vi "Option Selection.vi"(0 "GEA2 Reference In":refnum<k24>, 5 "Options":T2, 7 "Change":T1, 9 "Change All?":bool, 11 "Error In":errorcluster) -> (4 "GEA2 Reference Out":refnum<k24>, 15 "Error Out":errorcluster)   [LabVIEW 2016, in "2015 VA Washer.lvlib"]
doc: "Use this VI to select options on the HEUI or LEUI. These options are selected through their respective ERDs, not by a button press or knob turn."
uses:
  Projects/2015 VA Washer.lvlib
  C:/Automation/DLLs/PC Dot Net/GeaCommunication.dll
  Common/LabVIEW GEA2 Toolkit/LabVIEW_GEA2_Toolkit.lvlibp/type defs/Source_Destination.ctl
  Common/LabVIEW GEA2 Toolkit/LabVIEW_GEA2_Toolkit.lvlibp/type defs/ERD Write Data In.ctl
  Common/LabVIEW GEA2 Toolkit/LabVIEW_GEA2_Toolkit.lvlibp/type defs/Data Type.ctl
  Common/LabVIEW GEA2 Toolkit/LabVIEW_GEA2_Toolkit.lvlibp
panel:
  in  "Standalone?":bool
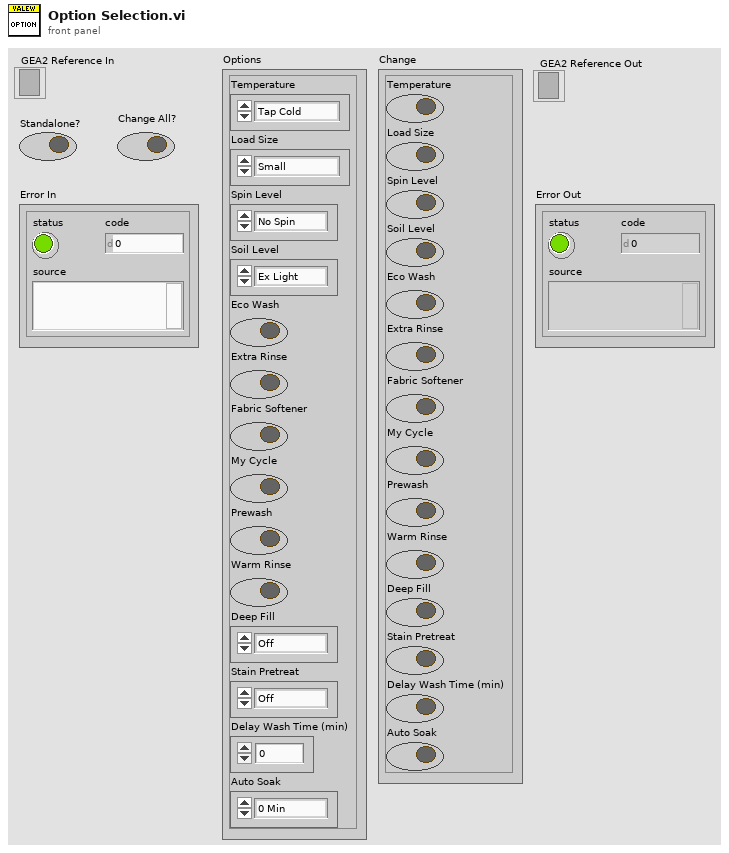
[diagram p1: front panel]
types:
  T1 = cluster{"Temperature":bool, "Load Size":bool, "Spin Level":bool, "Soil Level":bool, "Eco Wash":bool, "Extra Rinse":bool, "Fabric Softener":bool, "My Cycle":bool, "Prewash":bool, "Warm Rinse":bool, "Deep Fill":bool, "Stain Pretreat":bool, "Delay Wash Time (min)":bool, "Auto Soak":bool}
  T2 = cluster{"Temperature":enum16{"Tap Cold", "Cold", "Cool", "Colors", "Warm", "Hot"}, "Load Size":enum16{"Small", "Medium", "Large", "Super", "Precise Fill (Super Plus)"}, "Spin Level":enum16{"No Spin", "Normal", "More", "Max"}, "Soil Level":enum16{"Ex Light", "Light", "Normal", "Heavy", "Ex Heavy"}, "Eco Wash":bool, "Extra Rinse":bool, "Fabric Softener":bool, "My Cycle":bool, "Prewash":bool, "Warm Rinse":bool, "Deep Fill":enum16{"Off", "Incremental", "Max"}, "Stain Pretreat":enum16{"Off", "Tomato", "Wine", "Blood", "Grass", "Dirt"}, "Delay Wash Time (min)":u16, "Auto Soak":enum16{"0 Min", "15 Min", "30 Min", "60 Min", "2 Hr"}}
  T3 = typedef "LabVIEW_GEA2_Toolkit.lvlibp/Source_Destination.ctl" = cluster{"Source":u8, "Destination":u8}
  T4 = enum16{"Tap Cold", "Cold", "Cool", "Colors", "Warm", "Hot"}
  T5 = typedef "LabVIEW_GEA2_Toolkit.lvlibp/ERD Write Data In.ctl" = cluster{"ERD Number":u16, "Data Type":T6, "Data":string}
  T6 = typedef "LabVIEW_GEA2_Toolkit.lvlibp/Data Type.ctl" = enum16{"string", "boolean", "uint8_t", "uint16_t", "uint32_t", "uint64_t", "int8_t", "int16_t", "int32_t", "int64_t"}
  T7 = enum16{"Small", "Medium", "Large", "Super", "Precise Fill (Super Plus)"}
  T8 = enum16{"Ex Light", "Light", "Normal", "Heavy", "Ex Heavy"}
  T9 = enum16{"Off", "Tomato", "Wine", "Blood", "Grass", "Dirt"}
  T10 = enum16{"0 Min", "15 Min", "30 Min", "60 Min", "2 Hr"}
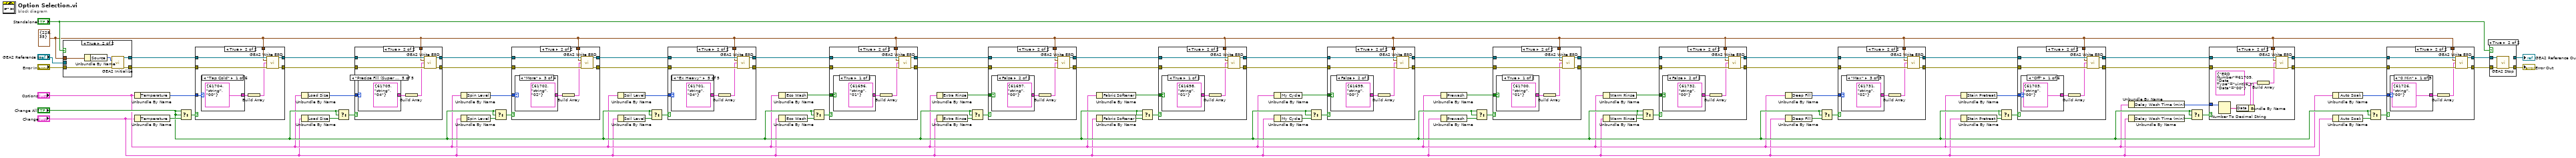
[diagram p0: block diagram]
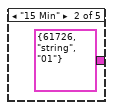
[diagram p4: hidden frame]
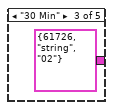
[diagram p5: hidden frame]
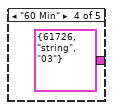
[diagram p6: hidden frame]
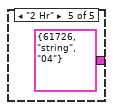
[diagram p7: hidden frame]
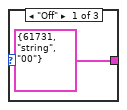
[diagram p9: hidden frame]
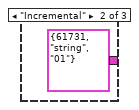
[diagram p10: hidden frame]
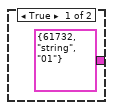
[diagram p12: hidden frame]
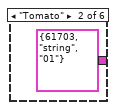
[diagram p14: hidden frame]
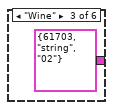
[diagram p15: hidden frame]
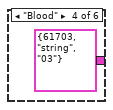
[diagram p16: hidden frame]
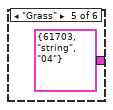
[diagram p17: hidden frame]
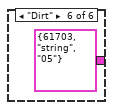
[diagram p18: hidden frame]
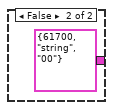
[diagram p20: hidden frame]
diagram:
  w8 = T3 {"Source"=228, "Destination"=35} ("GEA Inputs")
  n1 = case shown="True" "Standalone?" {
    tunnel: "Error In" -> [w82 w88]
    tunnel: [w82 w87] -> w76
    tunnel: "GEA2 Reference In" -> [w83 _]
    tunnel: [w83 w86] -> w81
    tunnel: w8 -> [_ w84]
    frame False {
    }
    frame True {
      n2 = Unbundle By Name(w84) -> ("Source"=w85:u8)
      n3 = call "GEA2 Initialize.vi"("Source Address"=w85, "error in"=w88) -> ("GEA2 Reference Out"=w86:refnum<k24>, "error out"=w87:errorcluster)  [unwired: 11 in, 1 out]
    }
  }
  n4 = Unbundle By Name("Options") -> ("Temperature"=w73:T4)
  n5 = Unbundle By Name("Change") -> ("Temperature"=w74:bool)
  n6 = Select(t="Change All?", s="Change All?", f=w74) -> (s? t:f=w72:bool)
  n7 = case shown="True" w72 {
    tunnel: w81 -> [w90 w98]
    tunnel: w76 -> [w89 w97]
    tunnel: w8 -> [_ w96]
    tunnel: [w90 w94] -> w68
    tunnel: [w89 w93] -> w67
    tunnel: w73 -> [_ w91]
    frame False {
    }
    frame True {
      n8 = case shown="\"Tap Cold\"" w91 {
        tunnel: [T5 {"ERD Number"=61704, "Data Type"=enum."string", "Data"="00"} ("ERD Write Data In") T5 {"ERD Number"=61704, "Data Type"=enum."string", "Data"="01"} ("ERD Write Data In") T5 {"ERD Number"=61704, "Data Type"=enum."string", "Data"="02"} ("ERD Write Data In") T5 {"ERD Number"=61704, "Data Type"=enum."string", "Data"="03"} ("ERD Write Data In") T5 {"ERD Number"=61704, "Data Type"=enum."string", "Data"="04"} ("ERD Write Data In") T5 {"ERD Number"=61704, "Data Type"=enum."string", "Data"="05"} ("ERD Write Data In")] -> w92
        frame "Tap Cold" {
        }
        frame "Cold" {
        }
        frame "Cool" {
        }
        frame "Colors" {
        }
        frame "Warm" {
        }
        frame "Hot" {
        }
      }
      n9 = Build Array(w92) -> (w95:T5[])
      n10 = call "GEA2 Write ERD.vi"("GEA2 Reference In"=w98, "GEA Inputs"=w96, "Write ERD List"=w95, "Error In"=w97) -> ("GEA2 Reference Out"=w94:refnum<k24>, "Error Out"=w93:errorcluster)  [unwired: 9 in, 1 out]
    }
  }
  n11 = Unbundle By Name("Options") -> ("Load Size"=w70:T7)
  n12 = Unbundle By Name("Change") -> ("Load Size"=w69:bool)
  n13 = Select(t="Change All?", s="Change All?", f=w69) -> (s? t:f=w71:bool)
  n14 = case shown="True" w71 {
    tunnel: w68 -> [w106 w114]
    tunnel: w67 -> [w105 w113]
    tunnel: w8 -> [_ w112]
    tunnel: [w106 w109] -> w63
    tunnel: [w105 w108] -> w62
    tunnel: w70 -> [_ w107]
    frame False {
    }
    frame True {
      n15 = case shown="\"Precise Fill (Super Plus)\"" w107 {
        tunnel: [T5 {"ERD Number"=61705, "Data Type"=enum."string", "Data"="00"} ("ERD Write Data In") T5 {"ERD Number"=61705, "Data Type"=enum."string", "Data"="01"} ("ERD Write Data In") T5 {"ERD Number"=61705, "Data Type"=enum."string", "Data"="02"} ("ERD Write Data In") T5 {"ERD Number"=61705, "Data Type"=enum."string", "Data"="03"} ("ERD Write Data In") T5 {"ERD Number"=61705, "Data Type"=enum."string", "Data"="04"} ("ERD Write Data In")] -> w111
        frame "Small" {
        }
        frame "Medium" {
        }
        frame "Large" {
        }
        frame "Super" {
        }
        frame "Precise Fill (Super Plus)" {
        }
      }
      n16 = Build Array(w111) -> (w110:T5[])
      n17 = call "GEA2 Write ERD.vi"("GEA2 Reference In"=w114, "GEA Inputs"=w112, "Write ERD List"=w110, "Error In"=w113) -> ("GEA2 Reference Out"=w109:refnum<k24>, "Error Out"=w108:errorcluster)  [unwired: 9 in, 1 out]
    }
  }
  n18 = Unbundle By Name("Options") -> ("Spin Level"=w65:enum16{"No Spin", "Normal", "More", "Max"})
  n19 = Unbundle By Name("Change") -> ("Spin Level"=w66:bool)
  n20 = Select(t="Change All?", s="Change All?", f=w66) -> (s? t:f=w64:bool)
  n21 = case shown="True" w64 {
    tunnel: w63 -> [w121 w129]
    tunnel: w62 -> [w120 w128]
    tunnel: w8 -> [_ w127]
    tunnel: [w121 w124] -> w58
    tunnel: [w120 w123] -> w57
    tunnel: w65 -> [_ w122]
    frame False {
    }
    frame True {
      n22 = case shown="\"More\"" w122 {
        tunnel: [T5 {"ERD Number"=61702, "Data Type"=enum."string", "Data"="00"} ("ERD Write Data In") T5 {"ERD Number"=61702, "Data Type"=enum."string", "Data"="01"} ("ERD Write Data In") T5 {"ERD Number"=61702, "Data Type"=enum."string", "Data"="02"} ("ERD Write Data In") T5 {"ERD Number"=61702, "Data Type"=enum."string", "Data"="03"} ("ERD Write Data In")] -> w126
        frame "No Spin" {
        }
        frame "Normal" {
        }
        frame "More" {
        }
        frame "Max" {
        }
      }
      n23 = Build Array(w126) -> (w125:T5[])
      n24 = call "GEA2 Write ERD.vi"("GEA2 Reference In"=w129, "GEA Inputs"=w127, "Write ERD List"=w125, "Error In"=w128) -> ("GEA2 Reference Out"=w124:refnum<k24>, "Error Out"=w123:errorcluster)  [unwired: 9 in, 1 out]
    }
  }
  n25 = Unbundle By Name("Options") -> ("Soil Level"=w60:T8)
  n26 = Unbundle By Name("Change") -> ("Soil Level"=w59:bool)
  n27 = Select(t="Change All?", s="Change All?", f=w59) -> (s? t:f=w61:bool)
  n28 = case shown="True" w61 {
    tunnel: w58 -> [w135 w143]
    tunnel: w57 -> [w134 w142]
    tunnel: w8 -> [_ w141]
    tunnel: [w135 w138] -> w53
    tunnel: [w134 w137] -> w52
    tunnel: w60 -> [_ w136]
    frame False {
    }
    frame True {
      n29 = case shown="\"Ex Heavy\"" w136 {
        tunnel: [T5 {"ERD Number"=61701, "Data Type"=enum."string", "Data"="00"} ("ERD Write Data In") T5 {"ERD Number"=61701, "Data Type"=enum."string", "Data"="01"} ("ERD Write Data In") T5 {"ERD Number"=61701, "Data Type"=enum."string", "Data"="02"} ("ERD Write Data In") T5 {"ERD Number"=61701, "Data Type"=enum."string", "Data"="03"} ("ERD Write Data In") T5 {"ERD Number"=61701, "Data Type"=enum."string", "Data"="04"} ("ERD Write Data In")] -> w140
        frame "Ex Light" {
        }
        frame "Light" {
        }
        frame "Normal" {
        }
        frame "Heavy" {
        }
        frame "Ex Heavy" {
        }
      }
      n30 = Build Array(w140) -> (w139:T5[])
      n31 = call "GEA2 Write ERD.vi"("GEA2 Reference In"=w143, "GEA Inputs"=w141, "Write ERD List"=w139, "Error In"=w142) -> ("GEA2 Reference Out"=w138:refnum<k24>, "Error Out"=w137:errorcluster)  [unwired: 9 in, 1 out]
    }
  }
  n32 = Unbundle By Name("Options") -> ("Eco Wash"=w55:bool)
  n33 = Unbundle By Name("Change") -> ("Eco Wash"=w56:bool)
  n34 = Select(t="Change All?", s="Change All?", f=w56) -> (s? t:f=w54:bool)
  n35 = case shown="True" w54 {
    tunnel: w53 -> [w150 w158]
    tunnel: w52 -> [w149 w157]
    tunnel: w8 -> [_ w156]
    tunnel: [w150 w153] -> w47
    tunnel: [w149 w152] -> w48
    tunnel: w55 -> [_ w151]
    frame False {
    }
    frame True {
      n36 = case shown="True" w151 {
        tunnel: [T5 {"ERD Number"=61696, "Data Type"=enum."string", "Data"="01"} ("ERD Write Data In") T5 {"ERD Number"=61696, "Data Type"=enum."string", "Data"="00"} ("ERD Write Data In")] -> w155
        frame True {
        }
        frame False {
        }
      }
      n37 = Build Array(w155) -> (w154:T5[])
      n38 = call "GEA2 Write ERD.vi"("GEA2 Reference In"=w158, "GEA Inputs"=w156, "Write ERD List"=w154, "Error In"=w157) -> ("GEA2 Reference Out"=w153:refnum<k24>, "Error Out"=w152:errorcluster)  [unwired: 9 in, 1 out]
    }
  }
  n39 = Unbundle By Name("Options") -> ("Extra Rinse"=w50:bool)
  n40 = Unbundle By Name("Change") -> ("Extra Rinse"=w49:bool)
  n41 = Select(t="Change All?", s="Change All?", f=w49) -> (s? t:f=w51:bool)
  n42 = case shown="True" w51 {
    tunnel: w47 -> [w162 w170]
    tunnel: w48 -> [w161 w169]
    tunnel: w8 -> [_ w168]
    tunnel: [w162 w165] -> w43
    tunnel: [w161 w164] -> w42
    tunnel: w50 -> [_ w163]
    frame False {
    }
    frame True {
      n43 = case shown="False" w163 {
        tunnel: [T5 {"ERD Number"=61697, "Data Type"=enum."string", "Data"="01"} ("ERD Write Data In") T5 {"ERD Number"=61697, "Data Type"=enum."string", "Data"="00"} ("ERD Write Data In")] -> w167
        frame True {
        }
        frame False {
        }
      }
      n44 = Build Array(w167) -> (w166:T5[])
      n45 = call "GEA2 Write ERD.vi"("GEA2 Reference In"=w170, "GEA Inputs"=w168, "Write ERD List"=w166, "Error In"=w169) -> ("GEA2 Reference Out"=w165:refnum<k24>, "Error Out"=w164:errorcluster)  [unwired: 9 in, 1 out]
    }
  }
  n46 = Unbundle By Name("Options") -> ("Fabric Softener"=w45:bool)
  n47 = Unbundle By Name("Change") -> ("Fabric Softener"=w46:bool)
  n48 = Select(t="Change All?", s="Change All?", f=w46) -> (s? t:f=w44:bool)
  n49 = case shown="True" w44 {
    tunnel: w43 -> [w174 w182]
    tunnel: w42 -> [w173 w181]
    tunnel: w8 -> [_ w180]
    tunnel: [w174 w177] -> w38
    tunnel: [w173 w176] -> w37
    tunnel: w45 -> [_ w175]
    frame False {
    }
    frame True {
      n50 = case shown="True" w175 {
        tunnel: [T5 {"ERD Number"=61698, "Data Type"=enum."string", "Data"="01"} ("ERD Write Data In") T5 {"ERD Number"=61698, "Data Type"=enum."string", "Data"="00"} ("ERD Write Data In")] -> w179
        frame True {
        }
        frame False {
        }
      }
      n51 = Build Array(w179) -> (w178:T5[])
      n52 = call "GEA2 Write ERD.vi"("GEA2 Reference In"=w182, "GEA Inputs"=w180, "Write ERD List"=w178, "Error In"=w181) -> ("GEA2 Reference Out"=w177:refnum<k24>, "Error Out"=w176:errorcluster)  [unwired: 9 in, 1 out]
    }
  }
  n53 = Unbundle By Name("Options") -> ("My Cycle"=w40:bool)
  n54 = Unbundle By Name("Change") -> ("My Cycle"=w39:bool)
  n55 = Select(t="Change All?", s="Change All?", f=w39) -> (s? t:f=w41:bool)
  n56 = case shown="True" w41 {
    tunnel: w38 -> [w186 w194]
    tunnel: w37 -> [w185 w193]
    tunnel: w8 -> [_ w192]
    tunnel: [w186 w189] -> w33
    tunnel: [w185 w188] -> w32
    tunnel: w40 -> [_ w187]
    frame False {
    }
    frame True {
      n57 = case shown="False" w187 {
        tunnel: [T5 {"ERD Number"=61699, "Data Type"=enum."string", "Data"="01"} ("ERD Write Data In") T5 {"ERD Number"=61699, "Data Type"=enum."string", "Data"="00"} ("ERD Write Data In")] -> w191
        frame True {
        }
        frame False {
        }
      }
      n58 = Build Array(w191) -> (w190:T5[])
      n59 = call "GEA2 Write ERD.vi"("GEA2 Reference In"=w194, "GEA Inputs"=w192, "Write ERD List"=w190, "Error In"=w193) -> ("GEA2 Reference Out"=w189:refnum<k24>, "Error Out"=w188:errorcluster)  [unwired: 9 in, 1 out]
    }
  }
  n60 = Unbundle By Name("Options") -> ("Prewash"=w35:bool)
  n61 = Unbundle By Name("Change") -> ("Prewash"=w36:bool)
  n62 = Select(t="Change All?", s="Change All?", f=w36) -> (s? t:f=w34:bool)
  n63 = case shown="True" w34 {
    tunnel: w33 -> [w198 w206]
    tunnel: w32 -> [w197 w205]
    tunnel: w8 -> [_ w204]
    tunnel: [w198 w201] -> w25
    tunnel: [w197 w200] -> w24
    tunnel: w35 -> [_ w199]
    frame False {
    }
    frame True {
      n64 = case shown="True" w199 {
        tunnel: [T5 {"ERD Number"=61700, "Data Type"=enum."string", "Data"="01"} ("ERD Write Data In") T5 {"ERD Number"=61700, "Data Type"=enum."string", "Data"="00"} ("ERD Write Data In")] -> w203
        frame True {
        }
        frame False {
        }
      }
      n65 = Build Array(w203) -> (w202:T5[])
      n66 = call "GEA2 Write ERD.vi"("GEA2 Reference In"=w206, "GEA Inputs"=w204, "Write ERD List"=w202, "Error In"=w205) -> ("GEA2 Reference Out"=w201:refnum<k24>, "Error Out"=w200:errorcluster)  [unwired: 9 in, 1 out]
    }
  }
  n67 = Unbundle By Name("Options") -> ("Warm Rinse"=w27:bool)
  n68 = Unbundle By Name("Change") -> ("Warm Rinse"=w26:bool)
  n69 = Select(t="Change All?", s="Change All?", f=w26) -> (s? t:f=w28:bool)
  n70 = case shown="True" w28 {
    tunnel: w25 -> [w210 w218]
    tunnel: w24 -> [w209 w217]
    tunnel: w8 -> [_ w216]
    tunnel: [w210 w213] -> w20
    tunnel: [w209 w212] -> w19
    tunnel: w27 -> [_ w211]
    frame False {
    }
    frame True {
      n71 = case shown="False" w211 {
        tunnel: [T5 {"ERD Number"=61732, "Data Type"=enum."string", "Data"="01"} ("ERD Write Data In") T5 {"ERD Number"=61732, "Data Type"=enum."string", "Data"="00"} ("ERD Write Data In")] -> w215
        frame True {
        }
        frame False {
        }
      }
      n72 = Build Array(w215) -> (w214:T5[])
      n73 = call "GEA2 Write ERD.vi"("GEA2 Reference In"=w218, "GEA Inputs"=w216, "Write ERD List"=w214, "Error In"=w217) -> ("GEA2 Reference Out"=w213:refnum<k24>, "Error Out"=w212:errorcluster)  [unwired: 9 in, 1 out]
    }
  }
  n74 = Unbundle By Name("Options") -> ("Deep Fill"=w22:enum16{"Off", "Incremental", "Max"})
  n75 = Unbundle By Name("Change") -> ("Deep Fill"=w23:bool)
  n76 = Select(t="Change All?", s="Change All?", f=w23) -> (s? t:f=w21:bool)
  n77 = case shown="True" w21 {
    tunnel: w20 -> [w222 w230]
    tunnel: w19 -> [w221 w229]
    tunnel: w8 -> [_ w228]
    tunnel: [w222 w225] -> w18
    tunnel: [w221 w224] -> w17
    tunnel: w22 -> [_ w223]
    frame False {
    }
    frame True {
      n78 = case shown="\"Max\"" w223 {
        tunnel: [T5 {"ERD Number"=61731, "Data Type"=enum."string", "Data"="00"} ("ERD Write Data In") T5 {"ERD Number"=61731, "Data Type"=enum."string", "Data"="01"} ("ERD Write Data In") T5 {"ERD Number"=61731, "Data Type"=enum."string", "Data"="02"} ("ERD Write Data In")] -> w227
        frame "Off" {
        }
        frame "Incremental" {
        }
        frame "Max" {
        }
      }
      n79 = Build Array(w227) -> (w226:T5[])
      n80 = call "GEA2 Write ERD.vi"("GEA2 Reference In"=w230, "GEA Inputs"=w228, "Write ERD List"=w226, "Error In"=w229) -> ("GEA2 Reference Out"=w225:refnum<k24>, "Error Out"=w224:errorcluster)  [unwired: 9 in, 1 out]
    }
  }
  n81 = Unbundle By Name("Options") -> ("Stain Pretreat"=w30:T9)
  n82 = Unbundle By Name("Change") -> ("Stain Pretreat"=w29:bool)
  n83 = Select(t="Change All?", s="Change All?", f=w29) -> (s? t:f=w31:bool)
  n84 = case shown="True" w31 {
    tunnel: w18 -> [w235 w243]
    tunnel: w17 -> [w234 w242]
    tunnel: w8 -> [_ w241]
    tunnel: [w235 w238] -> w7
    tunnel: [w234 w237] -> w6
    tunnel: w30 -> [_ w236]
    frame False {
    }
    frame True {
      n85 = case shown="\"Off\"" w236 {
        tunnel: [T5 {"ERD Number"=61703, "Data Type"=enum."string", "Data"="00"} ("ERD Write Data In") T5 {"ERD Number"=61703, "Data Type"=enum."string", "Data"="01"} ("ERD Write Data In") T5 {"ERD Number"=61703, "Data Type"=enum."string", "Data"="02"} ("ERD Write Data In") T5 {"ERD Number"=61703, "Data Type"=enum."string", "Data"="03"} ("ERD Write Data In") T5 {"ERD Number"=61703, "Data Type"=enum."string", "Data"="04"} ("ERD Write Data In") T5 {"ERD Number"=61703, "Data Type"=enum."string", "Data"="05"} ("ERD Write Data In")] -> w240
        frame "Off" {
        }
        frame "Tomato" {
        }
        frame "Wine" {
        }
        frame "Blood" {
        }
        frame "Grass" {
        }
        frame "Dirt" {
        }
      }
      n86 = Build Array(w240) -> (w239:T5[])
      n87 = call "GEA2 Write ERD.vi"("GEA2 Reference In"=w243, "GEA Inputs"=w241, "Write ERD List"=w239, "Error In"=w242) -> ("GEA2 Reference Out"=w238:refnum<k24>, "Error Out"=w237:errorcluster)  [unwired: 9 in, 1 out]
    }
  }
  n88 = Unbundle By Name("Options") -> ("Delay Wash Time (min)"=w13:u16)
  n89 = Unbundle By Name("Change") -> ("Delay Wash Time (min)"=w12:bool)
  n90 = Select(t="Change All?", s="Change All?", f=w12) -> (s? t:f=w14:bool)
  n91 = case shown="True" w14 {
    tunnel: w7 -> [w251 w261]
    tunnel: w6 -> [w250 w260]
    tunnel: w8 -> [_ w259]
    tunnel: [w251 w257] -> w15
    tunnel: [w250 w256] -> w16
    tunnel: w13 -> [_ w253]
    frame False {
    }
    frame True {
      n92 = Number To Decimal String(number=w253) -> (decimal integer string=w252:string)  [unwired: 1 in]
      n93 = Bundle By Name(cluster=T5 {"ERD Number"=61709, "Data Type"=enum."uint16_t", "Data"="00"} ("ERD Write Data In"), "Data"=w252) -> (w254:T5)
      n94 = Build Array(w254) -> (w258:T5[])
      n95 = call "GEA2 Write ERD.vi"("GEA2 Reference In"=w261, "GEA Inputs"=w259, "Write ERD List"=w258, "Error In"=w260) -> ("GEA2 Reference Out"=w257:refnum<k24>, "Error Out"=w256:errorcluster)  [unwired: 9 in, 1 out]
    }
  }
  n96 = Unbundle By Name("Options") -> ("Auto Soak"=w10:T10)
  n97 = Unbundle By Name("Change") -> ("Auto Soak"=w11:bool)
  n98 = Select(t="Change All?", s="Change All?", f=w11) -> (s? t:f=w9:bool)
  n99 = case shown="True" w9 {
    tunnel: w15 -> [w263 w271]
    tunnel: w16 -> [w262 w270]
    tunnel: w8 -> [_ w269]
    tunnel: [w263 w266] -> w2
    tunnel: [w262 w265] -> w1
    tunnel: w10 -> [_ w264]
    frame False {
    }
    frame True {
      n100 = case shown="\"0 Min\"" w264 {
        tunnel: [T5 {"ERD Number"=61726, "Data Type"=enum."string", "Data"="00"} ("ERD Write Data In") T5 {"ERD Number"=61726, "Data Type"=enum."string", "Data"="01"} ("ERD Write Data In") T5 {"ERD Number"=61726, "Data Type"=enum."string", "Data"="02"} ("ERD Write Data In") T5 {"ERD Number"=61726, "Data Type"=enum."string", "Data"="03"} ("ERD Write Data In") T5 {"ERD Number"=61726, "Data Type"=enum."string", "Data"="04"} ("ERD Write Data In")] -> w268
        frame "0 Min" {
        }
        frame "15 Min" {
        }
        frame "30 Min" {
        }
        frame "60 Min" {
        }
        frame "2 Hr" {
        }
      }
      n101 = Build Array(w268) -> (w267:T5[])
      n102 = call "GEA2 Write ERD.vi"("GEA2 Reference In"=w271, "GEA Inputs"=w269, "Write ERD List"=w267, "Error In"=w270) -> ("GEA2 Reference Out"=w266:refnum<k24>, "Error Out"=w265:errorcluster)  [unwired: 9 in, 1 out]
    }
  }
  n103 = case shown="True" "Standalone?" {
    tunnel: [w278 w281] -> w80
    tunnel: w2 -> [w277 w280]
    tunnel: w1 -> [w278 w279]
    tunnel: [w277 _] -> w75
    frame False {
    }
    frame True {
      n104 = call "GEA2 Stop.vi"("GEA2 Reference In"=w280, "Error In"=w279) -> ("Error Out"=w281:errorcluster)  [unwired: 13 in]
    }
  }
  "Error Out" <- w80
  "GEA2 Reference Out" <- w75
